vi "Image_dX_dY.vi"(0 "Camera":T1="Travcam") -> (1 "X Offset":dbl=-999.0 format="%.2f", 2 "Y Offset":dbl=-999.0 format="%.2f")   [LabVIEW 2015]
uses:
  Camera Server/Camera enum/Camera enum.ctl
  Anemometry Sub Vis/File/Setup_Filetype.ctl
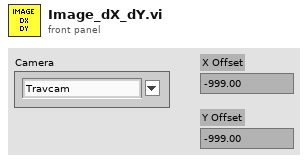
[diagram p1: front panel]
types:
  T1 = typedef "Camera enum.ctl" = string
  T2 = typedef "Setup_Filetype.ctl" = enum16{"Measurement Setups", "Calibration Setups", "General", "Results File Plotter Setups", "Speed Calib Tweaks"}
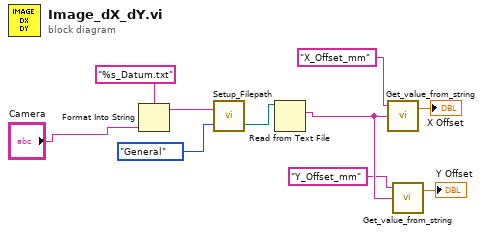
[diagram p0: block diagram]
diagram:
  n1 = Format Into String(format string="%s_Datum.txt", "Camera") -> (resulting string=w3:string)  [unwired: 2 in, 1 out]
  n2 = call "Setup_Filepath.vi"("Setup File Type"=Setup_Filetype."General", "Filename in"=w3) -> ("Filename Out"=w4:path)  [unwired: 1 out]
  n3 = Read from Text File(file (use dialog)=w4) -> (text=w7:string)  [unwired: 3 in, 3 out]
  n4 = call "Get_value_from_string.vi"("Input string"=w7, "Variable name"="X_Offset_mm") -> ("Value"=→"X Offset":dbl)  [unwired: 1 in, 1 out]
  n5 = call "Get_value_from_string.vi"("Input string"=w7, "Variable name"="Y_Offset_mm") -> ("Value"=→"Y Offset":dbl)  [unwired: 1 in, 1 out]
